vi "SmootherPath.vi"(4 "SameSmoothPath?":bool, 6 "ball":T1, 7 "Distances":dbl[](array[numeric]), 8 "Robot in":T2={"id"=0, "function"=enum."Attacker", "x"=0.0, "y"=0.0, "orientation"=0.0, "v_tangent"=0.0, "v_normal"=0.0, "v_ang"=0.0, "kick_x"=0.0, "kick_z"=0.0, "dribble"=FALSE, "Timestamp"=timestamp(0 s since 1904-01-01), "estimatives"={"est_v_tangent"=0.0, "est_v_normal"=0.0, "est_vx"=0.0, "est_vy"=0.0, "Pos Robot Est"=[]}, "dest_x_kick"=0.0, "dest_y_kick"=0.0, "Gap Coord"=[], "States"=enum."GoToTangent", "Path "=[], "Path  Smooth"=[], "Dest"=[]}, 9 "SmoothPath":dbl[][](array[numeric]), 10 "enemy_robots":T2[](array[typedef]), 11 "our_robots":T2[](array[typedef])) -> (1 "SmootherPath":dbl[][](array[numeric]), 3 "DistancesCalculated":dbl[](array[numeric]))   [LabVIEW 2017]
uses:
  Core/AI Robot.ctl
  Intel/Functions Enum.ctl
  Intel/AttackerStates.ctl
  PathDests.ctl
  PathDest.ctl
  Core/AI Ball.ctl
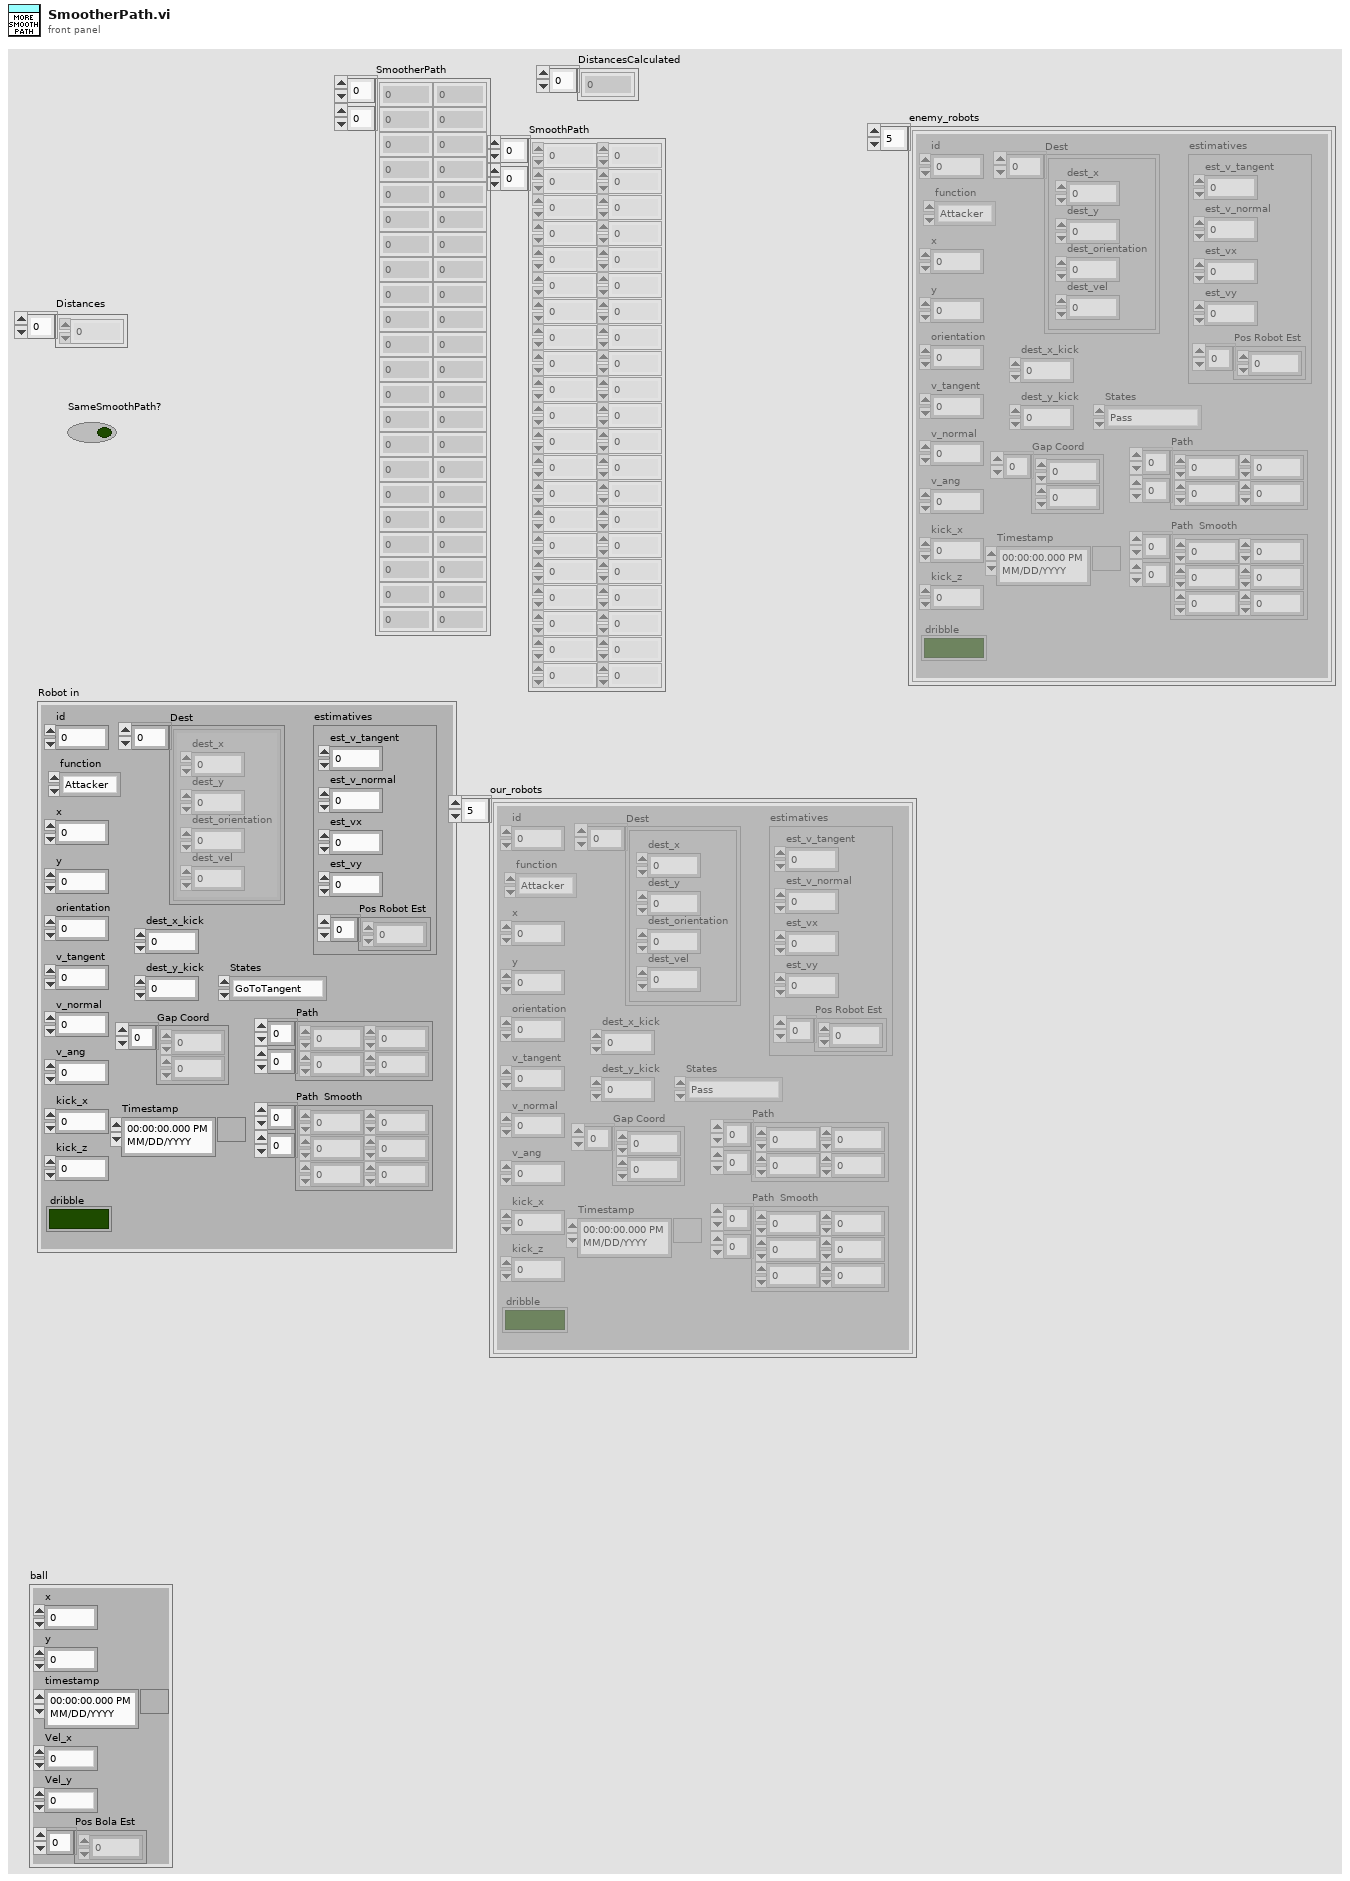
[diagram p1: front panel]
types:
  T1 = typedef "AI Ball.ctl" = cluster{"x":dbl, "y":dbl, "timestamp":timestamp, "Vel_x":dbl, "Vel_y":dbl, "Pos Bola Est":dbl[]}
  T2 = typedef "AI Robot.ctl" = cluster{"id":u32, "function":T3, "x":dbl, "y":dbl, "orientation":dbl, "v_tangent":dbl, "v_normal":dbl, "v_ang":dbl, "kick_x":dbl, "kick_z":dbl, "dribble":bool, "Timestamp":timestamp, "estimatives":cluster{"est_v_tangent":dbl, "est_v_normal":dbl, "est_vx":dbl, "est_vy":dbl, "Pos Robot Est":dbl[]}, "dest_x_kick":dbl, "dest_y_kick":dbl, "Gap Coord":dbl[], "States":T4, "Path ":dbl[][], "Path  Smooth":dbl[][], "Dest":T5}
  T3 = typedef "Functions Enum.ctl" = enum16{"Attacker", "Goalie", "Defender", "Striker", "Goto 0", "Dummy", "Kicker", "ZigZag"}
  T4 = typedef "AttackerStates.ctl" = enum16{"Pass", "GoToTangent", "BallGetting", "GoToKick", ""}
  T5 = typedef "PathDests.ctl" = T6[]
  T6 = typedef "PathDest.ctl" = cluster{"dest_x":dbl, "dest_y":dbl, "dest_orientation":dbl, "dest_vel":dbl}
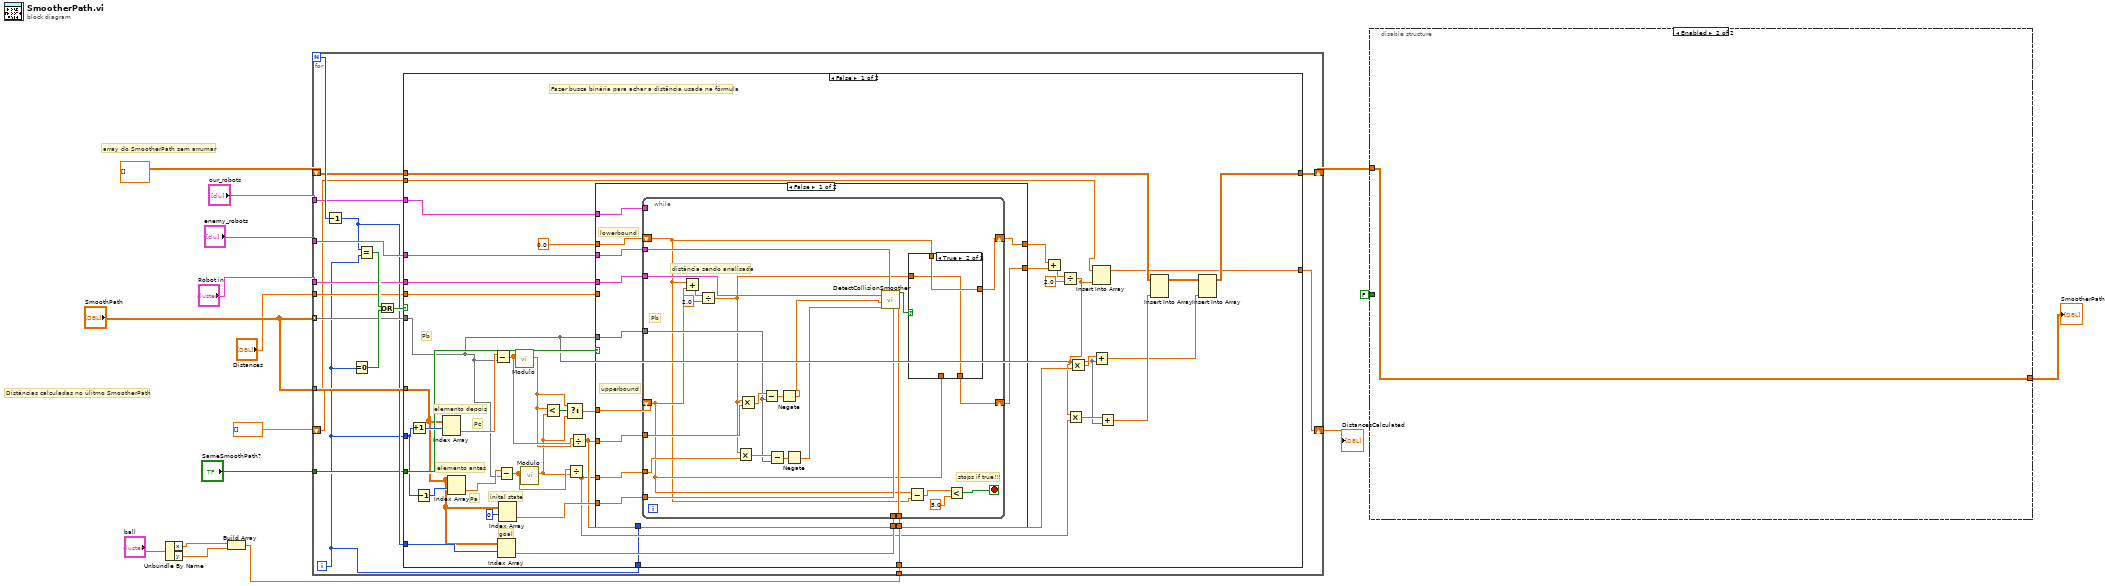
[diagram p0: block diagram]
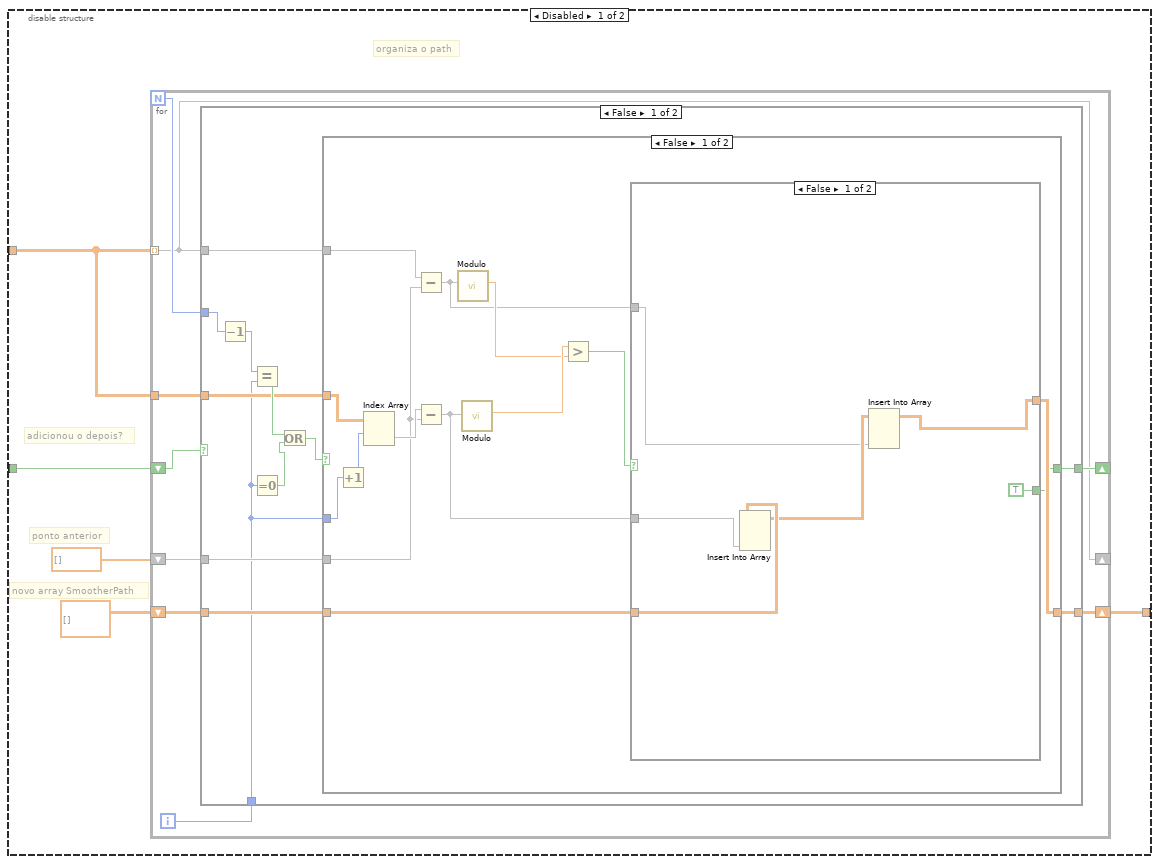
[diagram p2: hidden frame]
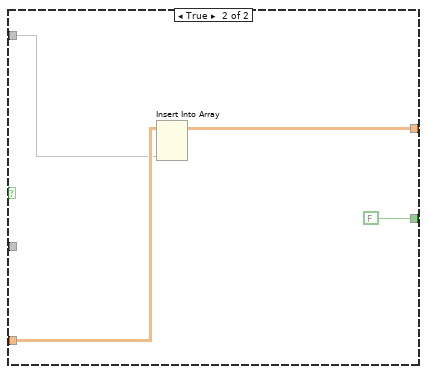
[diagram p3: hidden frame]
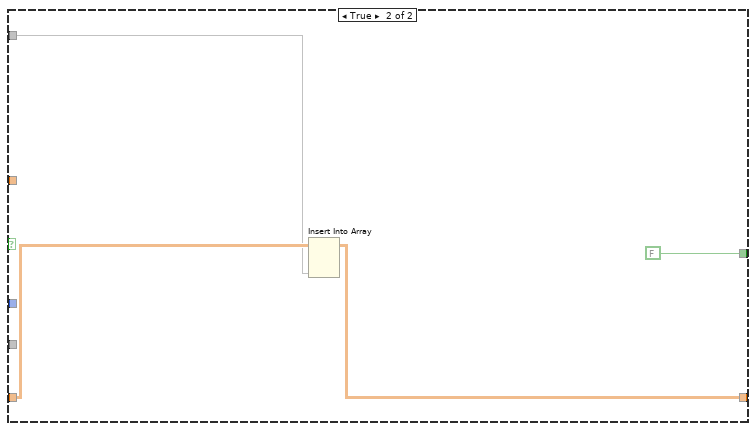
[diagram p4: hidden frame]
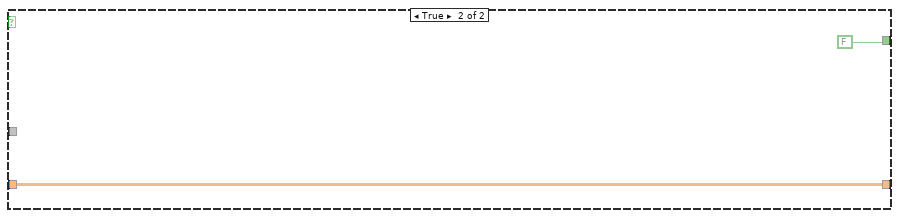
[diagram p5: hidden frame]
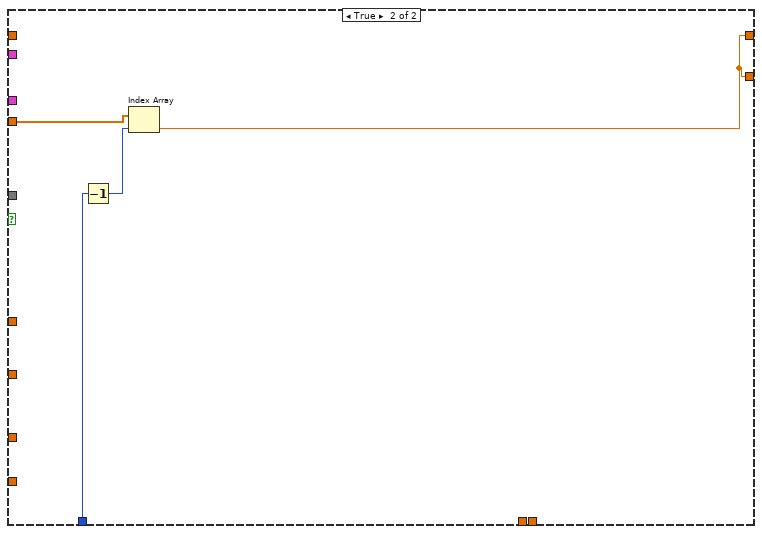
[diagram p7: hidden frame]
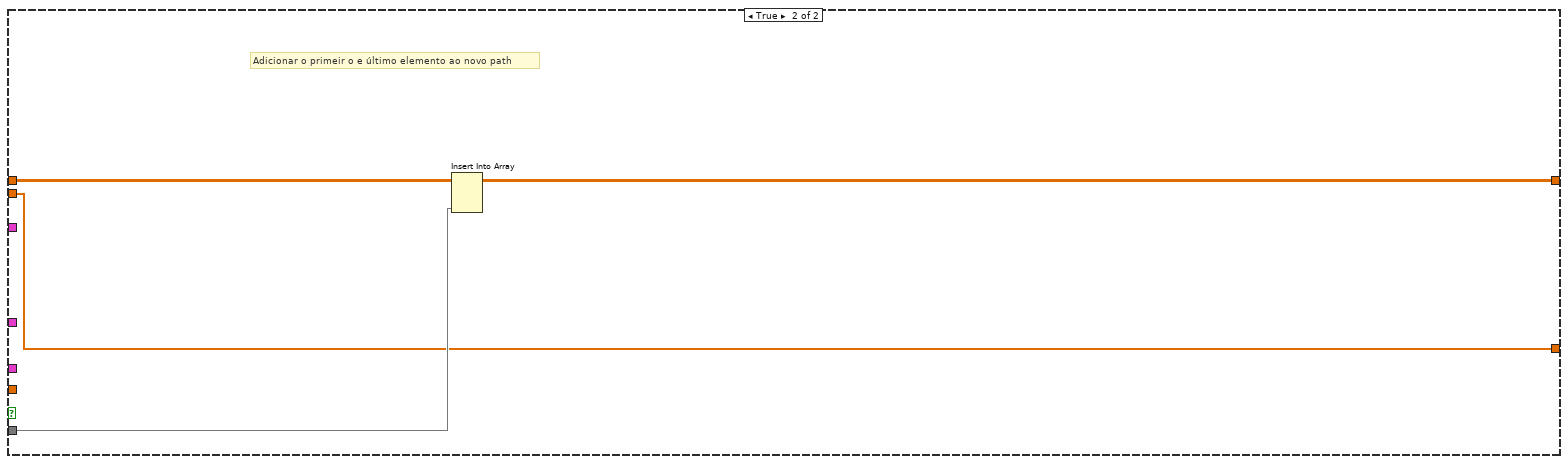
[diagram p8: hidden frame]
diagram:
  # "Distâncias calculadas no úlitmo SmootherPath"
  # "array do SmootherPath sem arrumar"
  n1 = Unbundle By Name("ball") -> ("x"=w15:dbl, "y"=w14:dbl)
  n2 = Build Array(w15, w14) -> (w9:dbl[])
  n3 = for {
    N -> [w34]
    tunnel: "SmoothPath" -> [w29] mode=indexing
    shift-right: [w28] -> w6
    shift-left: dbl[][] [] ("Path") -> [w31]
    tunnel: "SmoothPath" -> [w27]
    tunnel: "our_robots" -> [w26]
    tunnel: "enemy_robots" -> [w25]
    tunnel: "Robot in" -> [w24]
    tunnel: w9 -> [w22]
    tunnel: "SameSmoothPath?" -> [w21]
    tunnel: "Distances" -> [w20]
    shift-right: [w17] -> w1
    shift-left: dbl[] [] ("Distances") -> [w18]
    i -> [w19]
    n4 = Decrement(x=w34) -> (x-1=w23:i32)
    n5 = Equal To 0?(x=w19) -> (x = 0?=w32:bool)
    n6 = Equal?(x=w23, y=w19) -> (x = y?=w33:bool)
    n7 = Or(x=w33, y=w32) -> (x .or. y?=w30:bool)
    n8 = case shown="False" w30 {
      tunnel: w31 -> [w51 w124]
      tunnel: w29 -> [w38 w123]
      tunnel: [w49 w122] -> w28
      tunnel: w27 -> [w37 _]
      tunnel: w19 -> [w45 _]
      tunnel: w26 -> [w66 _]
      tunnel: w25 -> [w65 _]
      tunnel: w24 -> [w64 _]
      tunnel: w23 -> [w62 _]
      tunnel: w22 -> [w59 _]
      tunnel: w21 -> [w47 _]
      tunnel: w20 -> [w46 _]
      tunnel: w19 -> [w44 _]
      tunnel: w18 -> [w43 w121]
      tunnel: [w41 w121] -> w17
      frame False {
        # "Pa"
        # "Pc"
        # "Pb"
        # "goal"
        # "inital state"
        # "elemento antes"
        # "elemento depois"
        # "Fazer busca binária para achar a distãncia usada na fórmula"
        n9 = Increment(x=w45) -> (x+1=w75:i32)
        n10 = Decrement(x=w45) -> (x-1=w74:i32)
        n11 = Index Array(array=w37, index (row)=w75) -> (element=w40:dbl[])  [unwired: 1 in]
        n12 = Index Array(array=w37, index (row)=w74) -> (element=w39:dbl[])  [unwired: 1 in]
        n13 = Subtract(x=w40, y=w38) -> (x-y=w70:dbl[])
        n14 = Index Array(array=w37, index (row)=w62) -> (element=w60:dbl[])  [unwired: 1 in]
        n15 = Subtract(x=w39, y=w38) -> (x-y=w68:dbl[])
        n16 = Index Array(array=w37, index (row)=0) -> (element=w61:dbl[])  [unwired: 1 in]
        n17 = call "Modulo.vi"("2D vector"=w70) -> ("Modulo"=w69:dbl)  [unwired: 10 in]
        n18 = call "Modulo.vi"("2D vector"=w68) -> ("Modulo"=w67:dbl)  [unwired: 10 in]
        n19 = Less?(x=w69, y=w67) -> (x < y?=w72:bool)
        n20 = Select(t=w69, s=w72, f=w67) -> (s? t:f=w71:dbl)
        n21 = Divide(x=w68, y=w67) -> (x/y=w48:dbl[])
        n22 = Divide(x=w70, y=w69) -> (x/y=w52:dbl[])
        n23 = case shown="False" w47 {
          tunnel: 0.0 -> [w88 _]
          tunnel: w71 -> [w87 _]
          tunnel: w66 -> [w86 _]
          tunnel: w65 -> [w85 _]
          tunnel: w64 -> [w84 _]
          tunnel: w61 -> [w83 _]
          tunnel: w60 -> [w82 _]
          tunnel: w59 -> [w81 _]
          tunnel: [w80 w117] -> w56
          tunnel: [w79 w117] -> w55
          tunnel: w52 -> [w78 _]
          tunnel: w38 -> [w77 _]
          tunnel: w48 -> [w76 _]
          tunnel: w46 -> [_ w120]
          tunnel: w44 -> [_ w119]
          frame False {
            # "upperbound"
            # "lowerbound"
            n24 = while {
              shift-right: [w95] -> w80
              shift-left: w88 -> [w93]
              shift-right: [w94] -> w79
              shift-left: w87 -> [w96]
              tunnel: w77 -> [w103]
              tunnel: w76 -> [w107]
              tunnel: w78 -> [w106]
              tunnel: w86 -> [_]
              tunnel: w85 -> [w102]
              tunnel: w84 -> [w101]
              tunnel: w83 -> [w100]
              tunnel: w82 -> [w99]
              tunnel: w81 -> [_]
              stop <- w110 stop-if-true
              # "distância sendo analisada"
              # "Pb"
              # "stops if true!!!"
              n25 = Add(x=w93, y=w96) -> (x+y=w109:dbl)
              n26 = Divide(x=w109, y=2.0) -> (x/y=w97:dbl)
              n27 = Multiply(x=w97, y=w107) -> (x*y=w105:dbl[])
              n28 = Multiply(x=w97, y=w106) -> (x*y=w104:dbl[])
              n29 = Subtract(x=w104, y=w103) -> (x-y=w92:dbl[])
              n30 = Subtract(x=w105, y=w103) -> (x-y=w90:dbl[])
              n31 = Negate(x=w92) -> (-x=w91:dbl[])
              n32 = Negate(x=w90) -> (-x=w89:dbl[])
              n33 = call "DetectCollisionSmoother.vi"("Goal"=w99, "Initial State"=w100, "enemy_robots"=w102, "Robot in"=w101, "SegmentPointB"=w89, "SegmentPointA"=w91) -> ("Is there colision?"=w98:bool)  [unwired: 5 in]
              n34 = Subtract(x=w96, y=w93) -> (x-y=w112:dbl)
              n35 = case shown="True" w98 {
                tunnel: w97 -> [w114 w115]
                tunnel: w93 -> [_ w116]
                tunnel: w96 -> [w113 _]
                tunnel: [w114 w116] -> w95
                tunnel: [w113 w115] -> w94
                frame False {
                }
                frame True {
                }
              }
              n36 = Less?(x=w112, y=5.0) -> (x < y?=w110:bool)
            }
          }
          frame True {
            n37 = Decrement(x=w119) -> (x-1=w118:i32)
            n38 = Index Array(array=w120, index=w118) -> (element=w117:dbl)
          }
        }
        n39 = Add(x=w56, y=w55) -> (x+y=w58:dbl)
        n40 = Divide(x=w58, y=2.0) -> (x/y=w42:dbl)
        n41 = Multiply(x=w42, y=w48) -> (x*y=w54:dbl[])
        n42 = Multiply(x=w42, y=w52) -> (x*y=w53:dbl[])
        n43 = Insert Into Array(array=w43, new element=w42) -> (w41:dbl[])  [unwired: 1 in]
        n44 = Add(x=w53, y=w38) -> (x+y=w35:dbl[])
        n45 = Add(x=w54, y=w38) -> (x+y=w36:dbl[])
        n46 = Insert Into Array(array=w51, new element=w36) -> (w50:dbl[][])  [unwired: 2 in]
        n47 = Insert Into Array(array=w50, new element=w35) -> (w49:dbl[][])  [unwired: 2 in]
      }
      frame True {
        # "Adicionar o primeir o e último elemento ao novo path"
        n48 = Insert Into Array(array=w124, new element=w123) -> (w122:dbl[][])  [unwired: 2 in]
      }
    }
  }
  "DistancesCalculated" <- w1
  n49 = disable-structure shown="Enabled" {
    disable-tunnel: [w128 w181] -> w8
    disable-tunnel: FALSE -> [w127 _]
    disable-tunnel: w6 -> [w125 w181]
    frame Disabled {
      # "organiza o path"
      # "ponto anterior"
      # "novo array SmootherPath"
      # "adicionou o depois?"
      n50 = for {
        N -> [w137]
        shift-right: [w134] -> w128
        shift-left: dbl[][] [] ("Path") -> [w135]
        shift-right: [w133] -> _
        shift-left: w127 -> [w138]
        tunnel: w125 -> [w132] mode=indexing
        shift-right: [w132] -> _
        shift-left: dbl[] [] ("Path") -> [w131]
        tunnel: w125 -> [w130]
        i -> [w136]
        n51 = case shown="False" w138 {
          tunnel: w137 -> [w150 _]
          tunnel: w136 -> [w139 _]
          tunnel: w132 -> [w145 _]
          tunnel: w135 -> [w144 w180]
          tunnel: [w143 w180] -> w134
          tunnel: [w142 FALSE] -> w133
          tunnel: w131 -> [w141 _]
          tunnel: w130 -> [w140 _]
          frame False {
            n52 = Decrement(x=w150) -> (x-1=w149:i32)
            n53 = Equal?(x=w149, y=w139) -> (x = y?=w148:bool)
            n54 = Equal To 0?(x=w139) -> (x = 0?=w147:bool)
            n55 = Or(x=w148, y=w147) -> (x .or. y?=w146:bool)
            n56 = case shown="False" w146 {
              tunnel: w145 -> [w160 w177]
              tunnel: w144 -> [w155 w178]
              tunnel: [w153 w176] -> w143
              tunnel: [w152 FALSE] -> w142
              tunnel: w141 -> [w159 _]
              tunnel: w140 -> [w164 _]
              tunnel: w139 -> [w162 _]
              frame False {
                n57 = Increment(x=w162) -> (x+1=w163:i32)
                n58 = Index Array(array=w164, index (row)=w163) -> (element=w161:dbl[])  [unwired: 1 in]
                n59 = Subtract(x=w160, y=w159) -> (x-y=w154:dbl[])
                n60 = Subtract(x=w161, y=w159) -> (x-y=w151:dbl[])
                n61 = call "Modulo.vi"("2D vector"=w154) -> ("Modulo"=w156:dbl)  [unwired: 10 in]
                n62 = call "Modulo.vi"("2D vector"=w151) -> ("Modulo"=w158:dbl)  [unwired: 10 in]
                n63 = Greater?(x=w158, y=w156) -> (0:w157:bool)
                n64 = case shown="False" w157 {
                  tunnel: w155 -> [w169 w174]
                  tunnel: w154 -> [w167 w173]
                  tunnel: [w166 w172] -> w153
                  tunnel: [TRUE FALSE] -> w152
                  tunnel: w151 -> [w170 _]
                  frame False {
                    n65 = Insert Into Array(array=w169, new element=w170) -> (w168:dbl[][])  [unwired: 2 in]
                    n66 = Insert Into Array(array=w168, new element=w167) -> (w166:dbl[][])  [unwired: 2 in]
                  }
                  frame True {
                    n67 = Insert Into Array(array=w174, new element=w173) -> (w172:dbl[][])  [unwired: 2 in]
                  }
                }
              }
              frame True {
                n68 = Insert Into Array(array=w178, new element=w177) -> (w176:dbl[][])  [unwired: 2 in]
              }
            }
          }
          frame True {
          }
        }
      }
    }
    frame Enabled {
    }
  }
  "SmootherPath" <- w8
